vi "displayIndicatorElement.vi"(10 "viewThisComponent":refnum<class "ViewThisComponent.lvclass">) -> ()   [LabVIEW 2016, in "EXAViewElements.lvlib"]
doc: "Displays an indicator element."
uses:
  EXAViewElements.lvlib
  ViewThisComponent/ViewThisComponent.lvclass
  home/andres/ct_cmpuserevents/ComponentTemplateCore/ComponentModel/ComponentModel/View/View.lvclass
  ts_sallv_exa/DataTypes/logevent_DetailedState.ctl
  ComponentTemplateCore/ComponentModel/ComponentModel/View/View.lvclass
  ts_sallv_exa/SALLV_EXA.lvlib
panel:
  out "aMsdValue 3":dbl[unit] format="%.2f"
  out "aMsdValue 2":dbl[unit] format="%.2f"
  out "positionSettled":bool
  out "Measured Positions":T1(graph)
  out "aMsdValue":dbl[unit] format="%.2f"
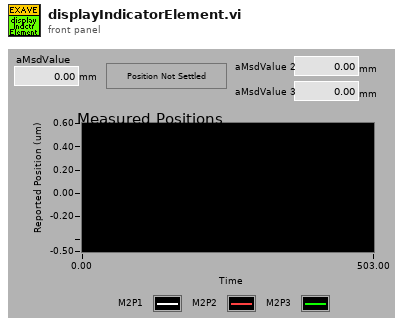
[diagram p1: front panel]
types:
  T1 = cluster{"Array of Double[0]":dbl, "Array of Double[1]":dbl, "Array of Double[2]":dbl}
  T2 = typedef "TypedefsDataEvents.lvlib/PubDataEvents.ctl" = cluster{"AppliedSettingsMatchStart":refnum<user-event>, "SettingVersions":refnum<user-event>, "SummaryState":refnum<user-event>, "RejectedCommand":refnum<user-event>, "DetailedState":refnum<user-event>, "ErrorCode":refnum<user-event>, "Heartbeat":refnum<user-event>, "LoopTime_ms":refnum<user-event>, "LoopTimeOutOfRange":refnum<user-event>, "Timestamp":refnum<user-event>}
  T3 = typedef "SALLV_EXA.lvlib/logevent_DetailedState.ctl" = cluster{"detailedState":enum16{"", " DisabledState", "EnabledState", "FaultState", "OfflineState", "StandbyState"}, "priority":i32}
  T4 = enum16{"", " DisabledState", "EnabledState", "FaultState", "OfflineState", "StandbyState"}
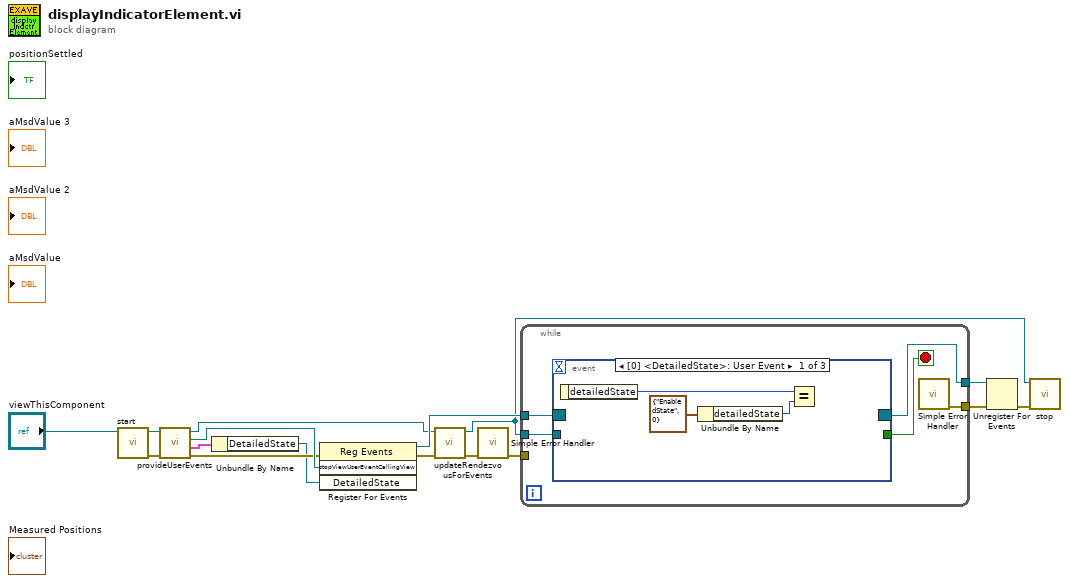
[diagram p0: block diagram]
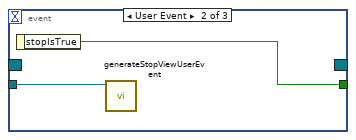
[diagram p2: hidden frame]
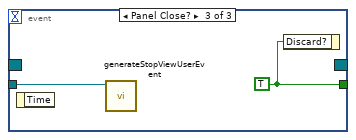
[diagram p3: hidden frame]
diagram:
  n1 = call-dynamic "start.vi"("View in"="viewThisComponent") -> ("error out"=w11:errorcluster, "View out"=w12:refnum<class "ViewThisComponent.lvclass">)  [unwired: 9 in]
  n2 = call "provideUserEvents.vi"("error in (no error)"=w11, "ViewThisComponent in"=w12) -> ("error out"=w13:errorcluster, "pubDataEvents"=w14:T2, "stopViewUserEventCallingView"=w15:refnum<user-event>, "ViewThisComponent out"=w2:refnum<class "ViewThisComponent.lvclass">)  [unwired: 6 in]
  n3 = Unbundle By Name(w14) -> ("DetailedState"=w10:refnum<user-event>)
  n4 = register-events(error in=w13, w15, w10) -> (reference out=w9:refnum<event-registration>, error out=w4:errorcluster)  [unwired: 1 in]
  n5 = call "updateRendezvousForEvents.vi"("error in (no error)"=w4, "View in"=w2) -> ("error out"=w3:errorcluster, "View out"=w1:refnum<class "ViewThisComponent.lvclass">)  [unwired: 8 in]
  n6 = call <vilib>:"Simple Error Handler.vi"("error in (no error)"=w3) -> ("error out"=w7:errorcluster)  [unwired: 4 in, 4 out]
  n7 = while {
    tunnel: w9 -> [w21]
    tunnel: w1 -> [w20]
    tunnel: [w19] -> w5
    tunnel: [w17] -> w8
    tunnel: w7 -> [_]
    stop <- w18 stop-if-true
    n8 = event shown="[0] <DetailedState>: User Event" {
      selector: w21 -> [_ _ _]
      dyn-events: [_ _ _] -> w17
      timeout: _ -> [_ _ _]
      tunnel: w20 -> [_ w25 w28]
      tunnel: [_ w26 w27] -> w18
      event User Event {
        n9 = event-data() -> ("detailedState"=w24:T4)  [unwired: 1 in]
        n10 = Unbundle By Name(T3 {"detailedState"=enum."EnabledState", "priority"=0} ("logevent_DetailedState")) -> ("detailedState"=w23:T4)
        n11 = Equal?(x=w24, y=w23) -> ()  [unwired: 1 out]
      }
      event User Event {
        n12 = event-data() -> ("stopIsTrue"=w26:bool)  [unwired: 1 in]
        n13 = call "generateStopViewUserEvent.vi"("View in"=w25) -> ()  [unwired: 9 in, 2 out]
      }
      event Panel Close? {
        w27 = TRUE ("Discard?")
        n14 = event-data() -> ()  [unwired: 1 in, 1 out]
        n15 = call "generateStopViewUserEvent.vi"("View in"=w28) -> ()  [unwired: 9 in, 2 out]
        n16 = event-data("Discard?"=w27) -> ()  [unwired: 1 in, 1 out]
      }
    }
    n17 = call <vilib>:"Simple Error Handler.vi"() -> ("error out"=w19:errorcluster)  [unwired: 5 in, 4 out]
  }
  n18 = Unregister For Events(event registration refnum=w8, error in=w5) -> (error out=w6:errorcluster)
  n19 = call-dynamic "stop.vi"("error in (no error)"=w6, "View in"=w1) -> ()  [unwired: 8 in, 2 out]
